vi "Main myRIO mirror.vi"() -> ()   [LabVIEW 2015]
panel:
  in  "TH":dbl
  out "Front-Left":bool
  out "Front-Right":bool
  out "Back Sensor":bool caption="Back"
  out "Tab Control":enum32{"Automaic", "Manual"}(tab)
  in  "GPS Port":refnum<visa-resource-name>
  out "Speed (KMPH)":dbl(slide) scale=0.0..100.0 scale format="%#_4g"
  out "GPS Signal":bool=TRUE
  out "Data Valid":bool=TRUE
  in  "Time Zone":i32=75
  out "Distacne to Go":T1
  out "Coordinates Out":T1
  out "Output":string
  in  "Control Type":bool
  in  "Command":T2(ring)
  in  "LED":bool
  in  "Stop 2":bool
  in  "Left":bool
  in  "Back":bool
  in  "Right":bool
  in  "Front":bool
  in  "Stop Button":bool
  out "Error Out":errorcluster
  out "Image":T3(plugin-control)
  in  "Stop":bool
  in  "Pause":bool
  in  "Start":bool
  in  "Claw Motor":u32(slide)=1548 scale=1400.0..1870.0
  in  "Elbow Motor":u32(slide)=2195 scale=1320.0..2290.0
  in  "Shoulder Motor":u32(slide)=730 scale=730.0..1490.0
  in  "Base Motor":u32(slide)=1300 scale=1300.0..2190.0
  out "Status":bool
  out "PIR":bool
  out "Morse In":bool
  in  "Morse Out":bool
  out "Y":i16
  out "X":i16
  out "BOOL O/P":T4
  out "CM O/P":cluster{"Back":sgl, "F-Left":sgl, "F-Right":sgl}
  # "Recon Rover Controls"
  # "Obstacle Sensor Readings"
  # "Image Stream"
  # "Arm Controls"
  # "Sensors"
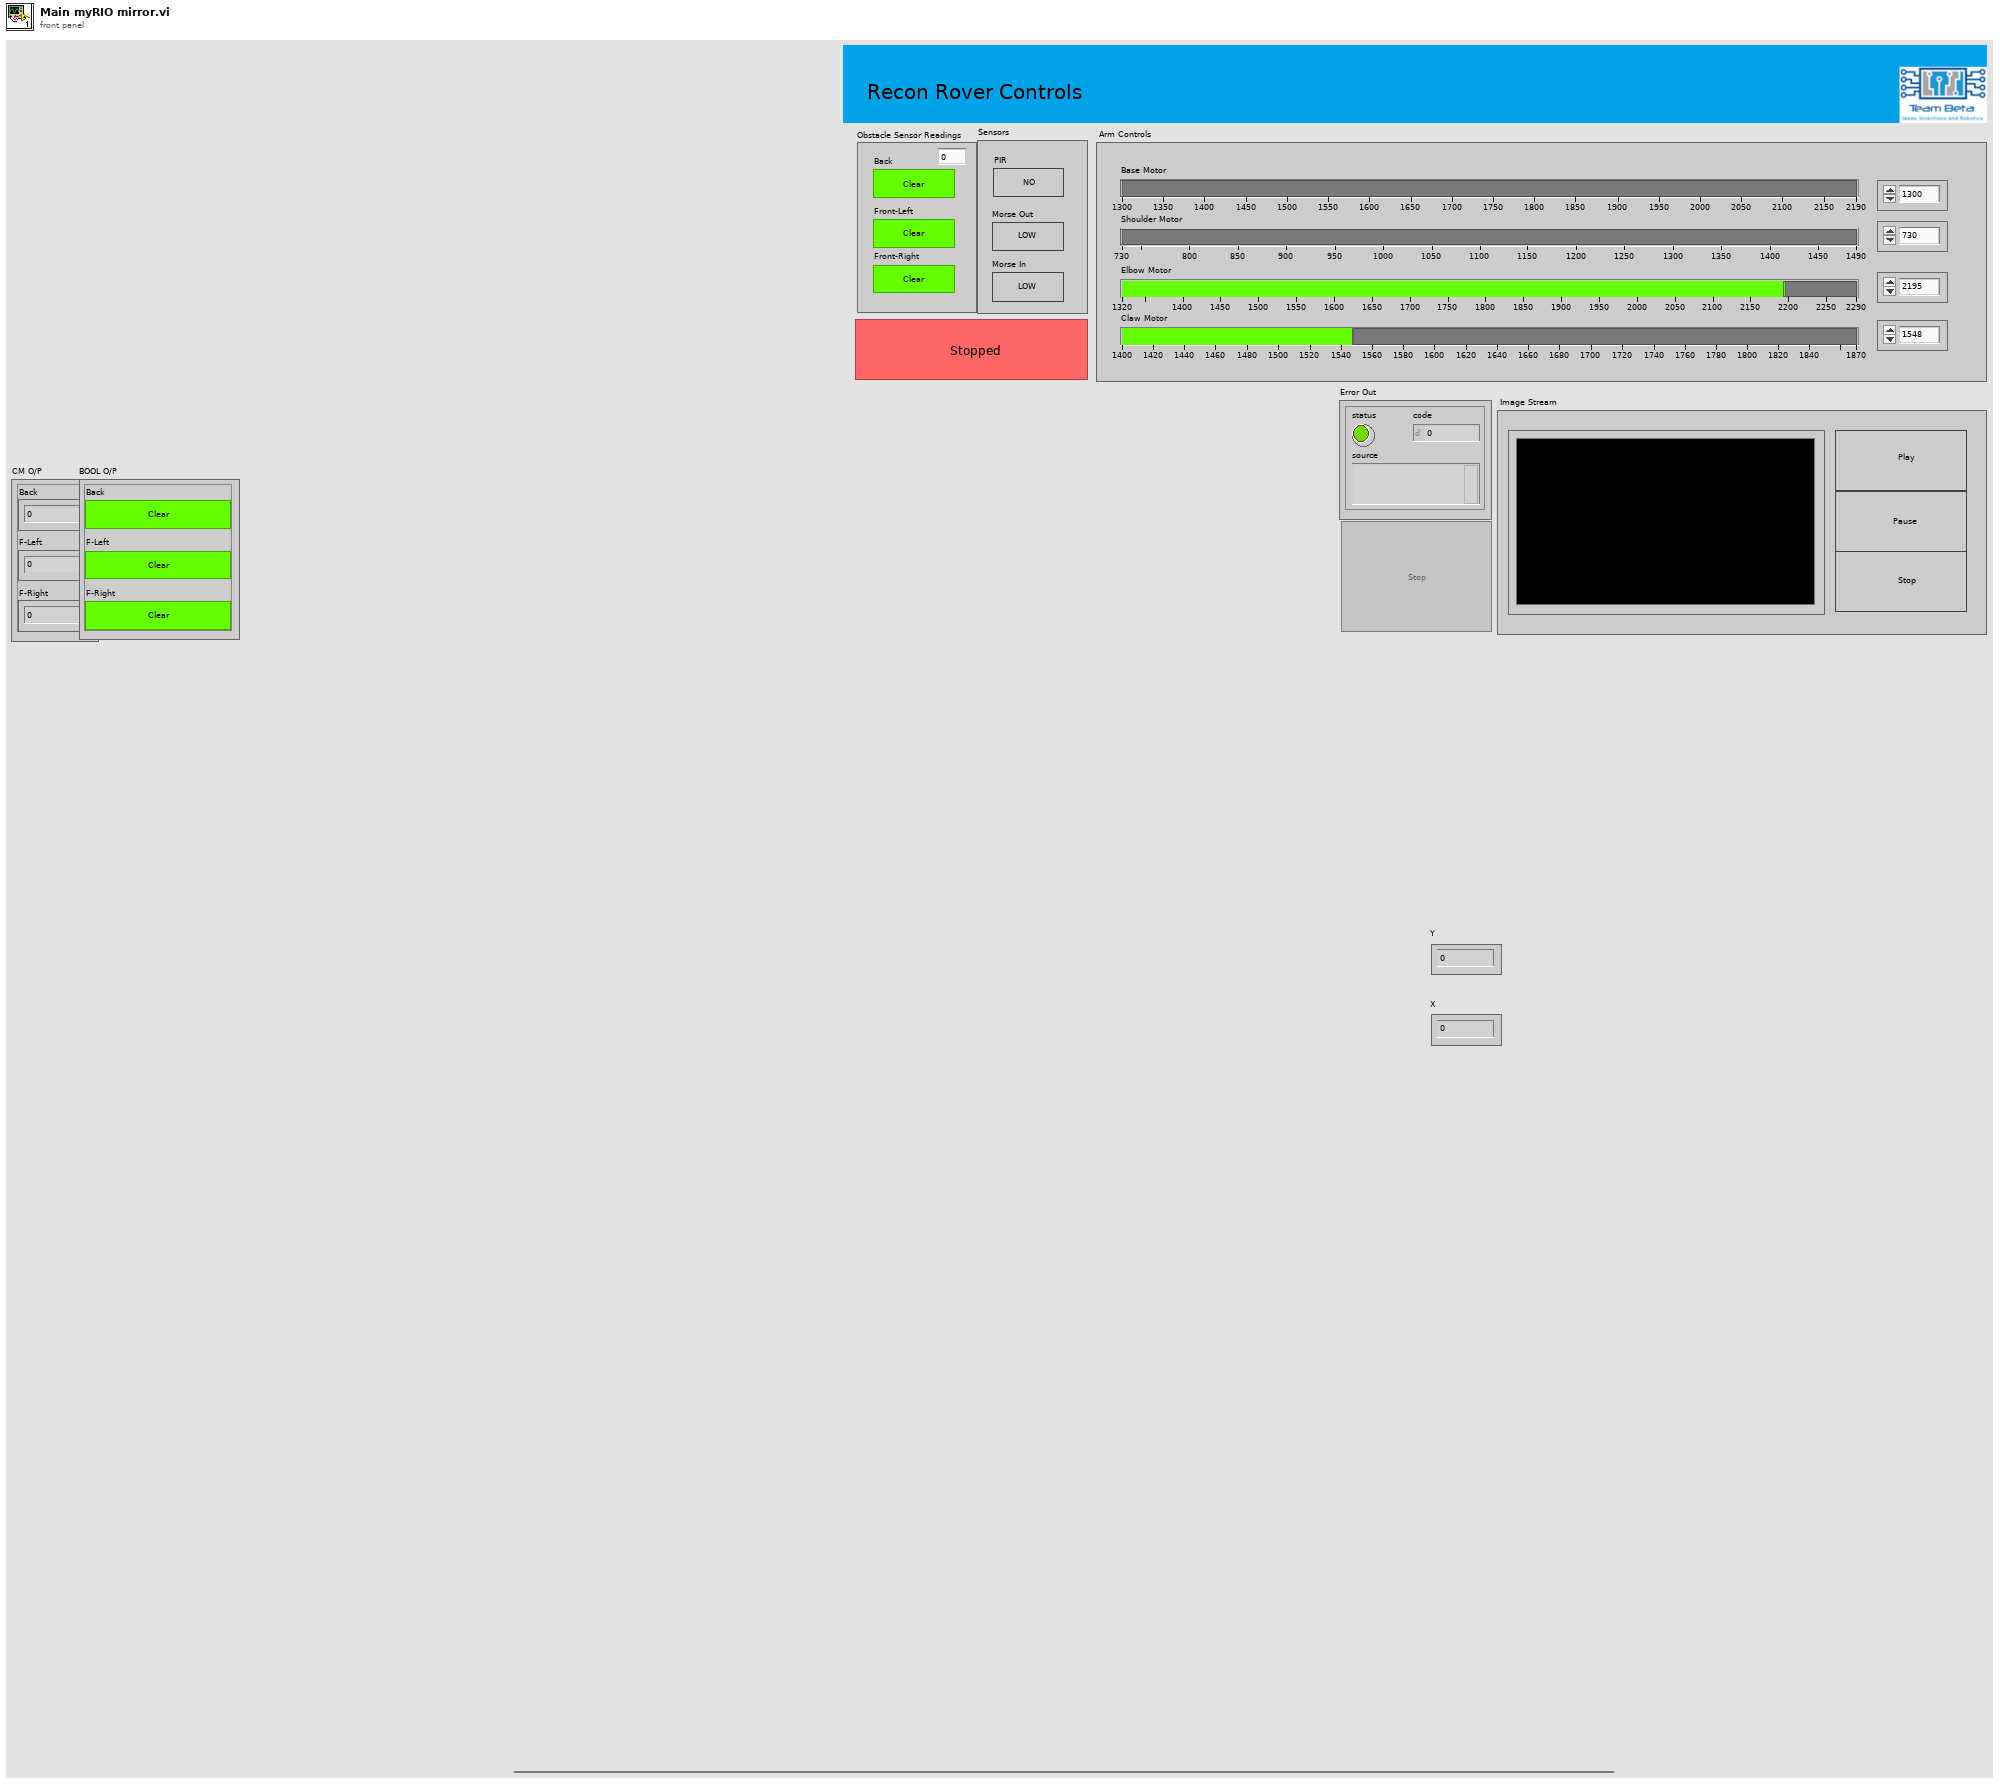
[diagram p1: front panel]
types:
  T1 = cluster{"Latitude":dbl, "Long":bool, "Longitude":dbl, "Lat":bool}
  T2 = enum16{"Stop", "LED", "Front", "Back", "Left", "Right"}
  T3 = typedef "IMAQ Image.ctl" = refnum<image>
  T4 = cluster{"Back":bool, "F-Right":bool, "F-Left":bool}
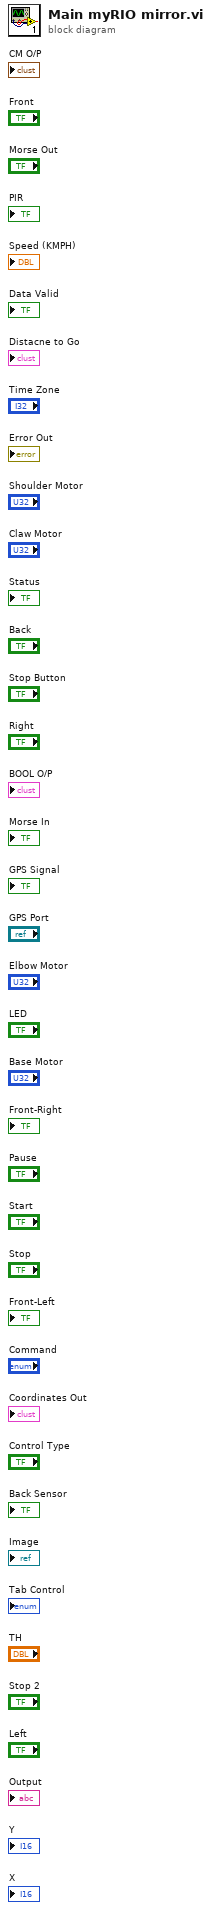
[diagram p0: block diagram]
diagram:
